vi "Rolling Display.vi"(6 "Input Data":dbl[][](array[numeric]), 8 "Channels in Use":T2, 9 "Old Data":dbl[][](array[numeric]), 10 "Sample Rate":i32, 11 "Display Size":T3(ring)) -> (1 "Array":dbl[][](array[numeric]), 3 "Cluster":T1)   [LabVIEW 2014]
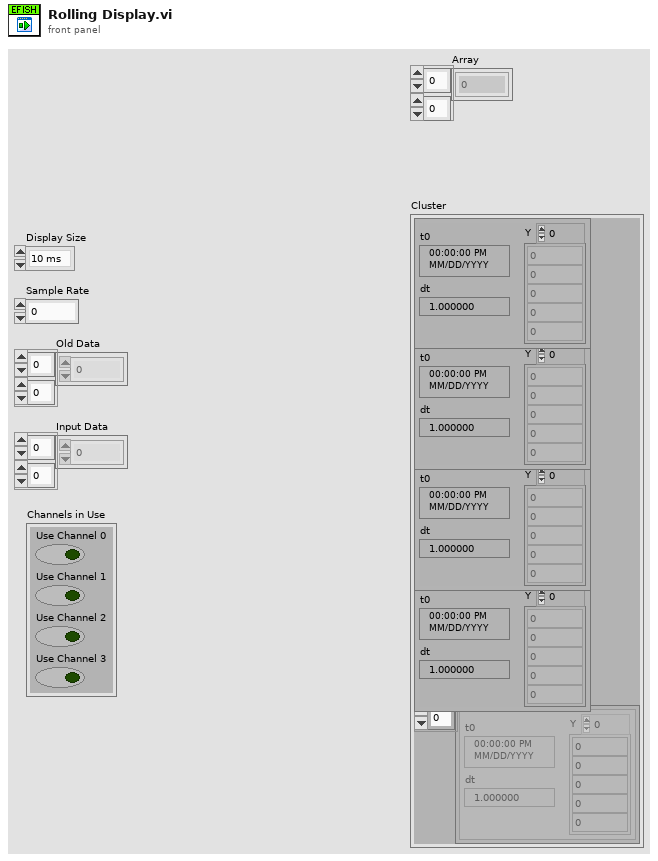
[diagram p1: front panel]
types:
  T1 = cluster{"Waveform":waveform(dbl), "Waveform":waveform(dbl), "Waveform":waveform(dbl), "Waveform":waveform(dbl), waveform(dbl)[]}
  T2 = cluster{"Use Channel 0":bool, "Use Channel 1":bool, "Use Channel 2":bool, "Use Channel 3":bool}
  T3 = enum16{"10 ms", "100 ms", "1 Second", "10 sec", "30 sec"}
  T4 = cluster{waveform(dbl), waveform(dbl), waveform(dbl), waveform(dbl), waveform(dbl)[]}
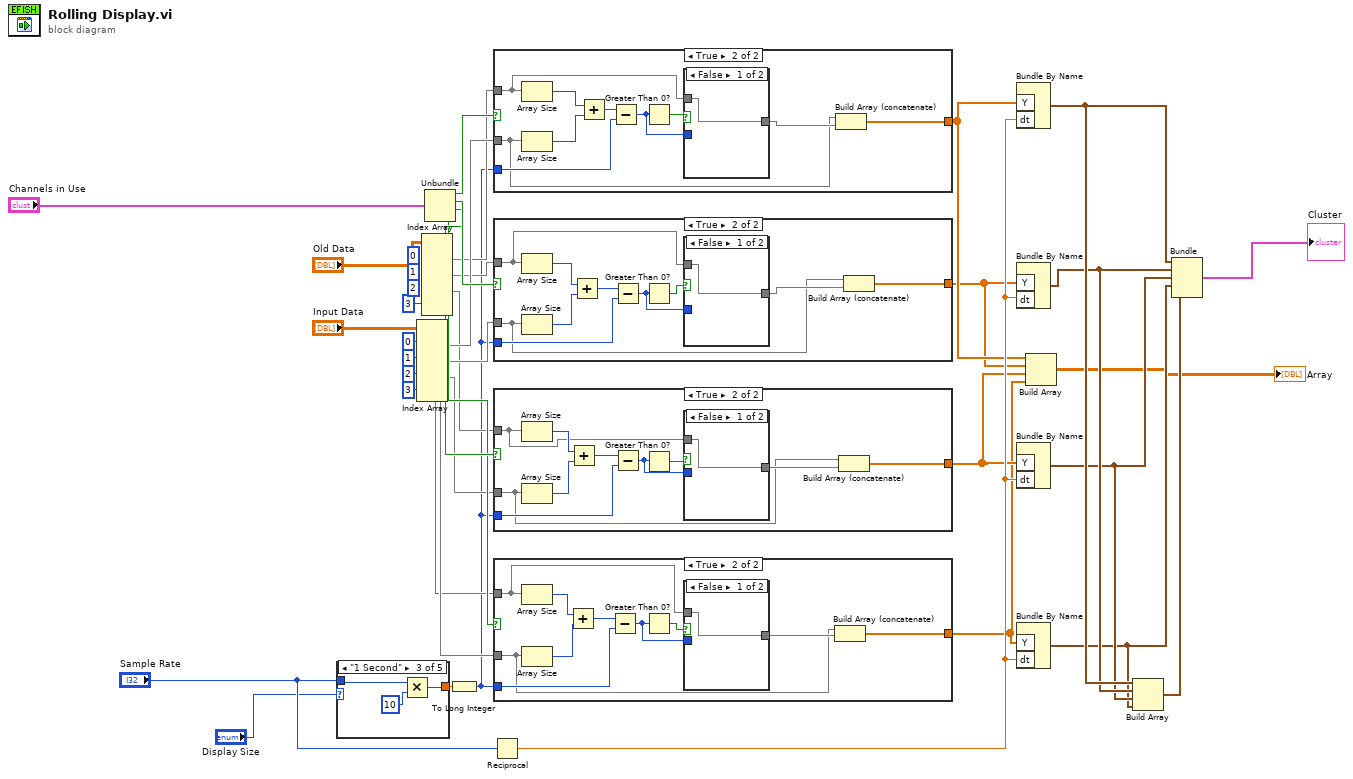
[diagram p0: block diagram]
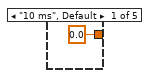
[diagram p2: hidden frame]
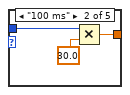
[diagram p3: hidden frame]
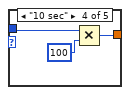
[diagram p4: hidden frame]
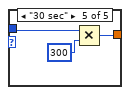
[diagram p5: hidden frame]
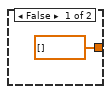
[diagram p6: hidden frame]
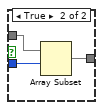
[diagram p7: hidden frame]
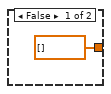
[diagram p8: hidden frame]
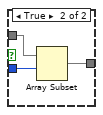
[diagram p9: hidden frame]
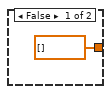
[diagram p10: hidden frame]
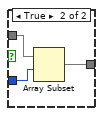
[diagram p11: hidden frame]
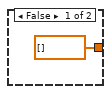
[diagram p12: hidden frame]
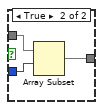
[diagram p13: hidden frame]
diagram:
  (unwired) 2 ("index (row)")
  (unwired) 1 ("index (row)")
  (unwired) 0 ("index (row)")
  n1 = case shown="\"1 Second\"" "Display Size" {
    tunnel: "Sample Rate" -> [_ w40 w42 w45 w48]
    tunnel: [0.0 w38 w43 w46 w49] -> w14
    frame "10 ms", Default {
    }
    frame "100 ms" {
      n2 = Multiply(x=w40, y=30.0) -> (x*y=w38:dbl)
    }
    frame "1 Second" {
      n3 = Multiply(x=w42, y=10) -> (x*y=w43:i32)
    }
    frame "10 sec" {
      n4 = Multiply(x=w45, y=100) -> (x*y=w46:i32)
    }
    frame "30 sec" {
      n5 = Multiply(x=w48, y=300) -> (x*y=w49:i32)
    }
  }
  n6 = Index Array(array="Input Data", index (row) #1=0 ("index (row)"), index (row) #2=1 ("index (row)"), index (row) #3=2 ("index (row)"), index (row) #4=3 ("index (row)")) -> (element #1=w23:dbl[], element #2=w22:dbl[], element #3=w21:dbl[], element #4=w20:dbl[])  [unwired: 4 in]
  n7 = Index Array(array="Old Data", index (row) #4=3 ("index (row)")) -> (element #1=w18:dbl[], element #2=w17:dbl[], element #3=w16:dbl[], element #4=w15:dbl[])  [unwired: 7 in]
  n8 = Unbundle("Channels in Use") -> ("Use Channel 0"=w31:bool, "Use Channel 1"=w30:bool, "Use Channel 2"=w29:bool, "Use Channel 3"=w28:bool)
  n9 = To Long Integer(number=w14) -> (32bit integer=w13:i32)
  n10 = Reciprocal(x="Sample Rate") -> (1/x=w12:dbl)
  n11 = case shown="True" w31 {
    tunnel: w23 -> [_ w52]
    tunnel: w18 -> [_ w54]
    tunnel: w13 -> [_ w57]
    tunnel: [dbl[] [] w51] -> w6
    frame False {
    }
    frame True {
      n12 = Array Size(array=w54) -> (size(s)=w60:i32)
      n13 = Array Size(array=w52) -> (size(s)=w59:i32)
      n14 = Add(x=w60, y=w59) -> (x+y=w58:i32)
      n15 = Subtract(x=w58, y=w57) -> (x-y=w55:i32)
      n16 = Greater Than 0?(x=w55) -> (x > 0?=w56:bool)
      n17 = case shown="False" w56 {
        tunnel: w55 -> [_ w64]
        tunnel: w54 -> [w61 w63]
        tunnel: [w61 w62] -> w53
        frame False {
        }
        frame True {
          n18 = Array Subset(array=w63, index=w64) -> (w62:dbl[])  [unwired: 1 in]
        }
      }
      n19 = Build Array (concatenate)(w52, w53) -> (w51:dbl[])
    }
  }
  n20 = case shown="True" w30 {
    tunnel: w22 -> [_ w67]
    tunnel: w17 -> [_ w69]
    tunnel: w13 -> [_ w72]
    tunnel: [dbl[] [] w66] -> w5
    frame False {
    }
    frame True {
      n21 = Array Size(array=w69) -> (size(s)=w75:i32)
      n22 = Array Size(array=w67) -> (size(s)=w74:i32)
      n23 = Add(x=w75, y=w74) -> (x+y=w73:i32)
      n24 = Subtract(x=w73, y=w72) -> (x-y=w70:i32)
      n25 = Greater Than 0?(x=w70) -> (x > 0?=w71:bool)
      n26 = case shown="False" w71 {
        tunnel: w70 -> [_ w79]
        tunnel: w69 -> [w76 w78]
        tunnel: [w76 w77] -> w68
        frame False {
        }
        frame True {
          n27 = Array Subset(array=w78, index=w79) -> (w77:dbl[])  [unwired: 1 in]
        }
      }
      n28 = Build Array (concatenate)(w67, w68) -> (w66:dbl[])
    }
  }
  n29 = case shown="True" w29 {
    tunnel: w21 -> [_ w82]
    tunnel: w16 -> [_ w84]
    tunnel: w13 -> [_ w87]
    tunnel: [dbl[] [] w81] -> w4
    frame False {
    }
    frame True {
      n30 = Array Size(array=w84) -> (size(s)=w90:i32)
      n31 = Array Size(array=w82) -> (size(s)=w89:i32)
      n32 = Add(x=w90, y=w89) -> (x+y=w88:i32)
      n33 = Subtract(x=w88, y=w87) -> (x-y=w85:i32)
      n34 = Greater Than 0?(x=w85) -> (x > 0?=w86:bool)
      n35 = case shown="False" w86 {
        tunnel: w85 -> [_ w94]
        tunnel: w84 -> [w91 w93]
        tunnel: [w91 w92] -> w83
        frame False {
        }
        frame True {
          n36 = Array Subset(array=w93, index=w94) -> (w92:dbl[])  [unwired: 1 in]
        }
      }
      n37 = Build Array (concatenate)(w82, w83) -> (w81:dbl[])
    }
  }
  n38 = case shown="True" w28 {
    tunnel: w20 -> [_ w97]
    tunnel: w15 -> [_ w99]
    tunnel: w13 -> [_ w102]
    tunnel: [dbl[] [] w96] -> w3
    frame False {
    }
    frame True {
      n39 = Array Size(array=w99) -> (size(s)=w105:i32)
      n40 = Array Size(array=w97) -> (size(s)=w104:i32)
      n41 = Add(x=w105, y=w104) -> (x+y=w103:i32)
      n42 = Subtract(x=w103, y=w102) -> (x-y=w100:i32)
      n43 = Greater Than 0?(x=w100) -> (x > 0?=w101:bool)
      n44 = case shown="False" w101 {
        tunnel: w100 -> [_ w109]
        tunnel: w99 -> [w106 w108]
        tunnel: [w106 w107] -> w98
        frame False {
        }
        frame True {
          n45 = Array Subset(array=w108, index=w109) -> (w107:dbl[])  [unwired: 1 in]
        }
      }
      n46 = Build Array (concatenate)(w97, w98) -> (w96:dbl[])
    }
  }
  n47 = Bundle By Name("Y"=w6, "dt"=w12) -> (w11:waveform(dbl))  [unwired: 1 in]
  n48 = Bundle By Name("Y"=w5, "dt"=w12) -> (w10:waveform(dbl))  [unwired: 1 in]
  n49 = Bundle By Name("Y"=w4, "dt"=w12) -> (w9:waveform(dbl))  [unwired: 1 in]
  n50 = Bundle By Name("Y"=w3, "dt"=w12) -> (w8:waveform(dbl))  [unwired: 1 in]
  n51 = Build Array(w6, w5, w4, w3) -> (→"Array":dbl[][])
  n52 = Build Array(w11, w10, w9, w8) -> (w7:waveform(dbl)[])
  n53 = Bundle(w11, w10, w9, w8, w7) -> (→"Cluster":T4)  [unwired: 1 in]
